vi "oa_FIR Param Change Check.vi"(7 "fs in [Hz]":dbl=1.0 format="%0.2f", 8 "filter type in":T2(ring), 10 "ripple specs in [dB]":cluster{"pass band":dbl, "stop band":dbl}={"pass band"=0.1, "stop band"=60.0} {"stop band" format="%0.2f"; "pass band" format="%0.2f"}, 11 "freq specs in [Hz]":T1={"fpass 1"=0.125, "fstop 1"=0.45, "fpass 2"=0.125, "fstop 2"=0.45} {"fstop 2" format="%0.2f"; "fpass 2" format="%.3f"; "fstop 1" format="%0.2f"; "fpass 1" format="%.3f"}) -> (0 "fs out":dbl=1.0 format="%0.2f", 2 "ripple specs out [dB]":cluster{"pass band":dbl, "stop band":dbl}, 3 "freq specs out [Hz]":T1, 4 "chang?":bool, 5 "filter type out":T2(ring))   [LabVIEW 2017, in "SoundVib_RefDataProcess.lvlib"]
uses:
  <vilib>/addons/Sound and Vibration/Order Analysis/Referece Data Processing/SoundVib_RefDataProcess.lvlib
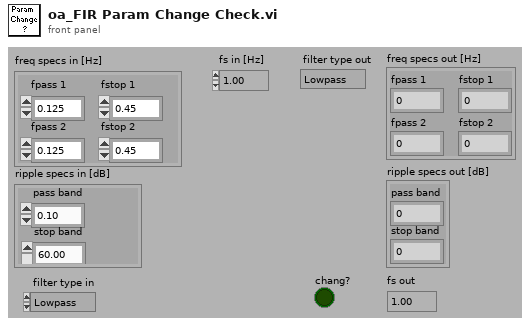
[diagram p1: front panel]
types:
  T1 = cluster{"fpass 1":dbl, "fstop 1":dbl, "fpass 2":dbl, "fstop 2":dbl}
  T2 = enum32{"Lowpass", "Highpass", "Bandpass", "Bandstop"}
  T3 = cluster{"fpass 1":bool, "fstop 1":bool, "fpass 2":bool, "fstop 2":bool}
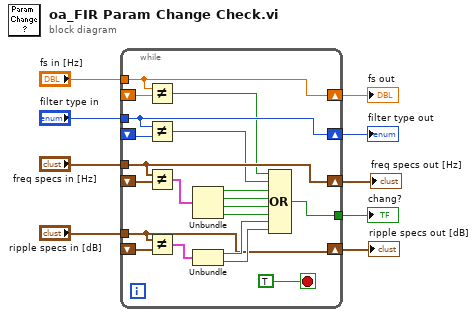
[diagram p0: block diagram]
diagram:
  n1 = while {
    tunnel: "fs in [Hz]" -> [w27]
    shift-right: [w27] -> w8
    shift-left: _ -> [w28]
    tunnel: "filter type in" -> [w26]
    shift-right: [w22] -> w2
    shift-left: _ -> [w23]
    shift-right: [w10] -> w1
    shift-left: _ -> [w19]
    shift-right: [w26] -> w7
    shift-left: _ -> [w25]
    tunnel: [w24] -> w3
    tunnel: "freq specs in [Hz]" -> [w22]
    tunnel: "ripple specs in [dB]" -> [w10]
    stop <- TRUE stop-if-true
    n2 = Not Equal?(x=w27, y=w28) -> (x != y?=w17:bool)
    n3 = Not Equal?(x=w26, y=w25) -> (x != y?=w18:bool)
    n4 = Not Equal?(x=w22, y=w23) -> (x != y?=w21:T3)
    n5 = Not Equal?(x=w10, y=w19) -> (x != y?=w20:cluster{"pass band":bool, "stop band":bool})
    n6 = Unbundle(w21) -> ("fpass 1"=w16:bool, "fstop 1"=w15:bool, "fpass 2"=w14:bool, "fstop 2"=w13:bool)
    n7 = Unbundle(w20) -> ("pass band"=w12:bool, "stop band"=w11:bool)
    n8 = Compound Arithmetic op=OR(w17, w18, w16, w15, w14, w13, w12, w11) -> (w24:bool)
  }
  "fs out" <- w8
  "filter type out" <- w7
  "chang?" <- w3
  "freq specs out [Hz]" <- w2
  "ripple specs out [dB]" <- w1
